vi "Scale Image.vi"(0 "ImageHandler in":refnum<class "ImageHandler.lvclass">, 5 "ImageIn":T1, 7 "Scale?":bool, 11 "error in":errorcluster, 12 "Max":i32, 13 "Min":i32) -> (4 "ImageHandler out":refnum<class "ImageHandler.lvclass">, 6 "ImageOut":T1, 15 "error out":errorcluster)   [LabVIEW 2022 SP3, in "ImageHandler.lvlib" / "ImageHandler.lvclass"]
uses:
  ImageHandler.lvclass
  <vilib>/vision/Image Controls.llb/IMAQ Image.ctl
  ImageHandler.lvclass/ImageHandler.ctl
  <vilib>/vision/NI_Vision_Development_Module.lvlib
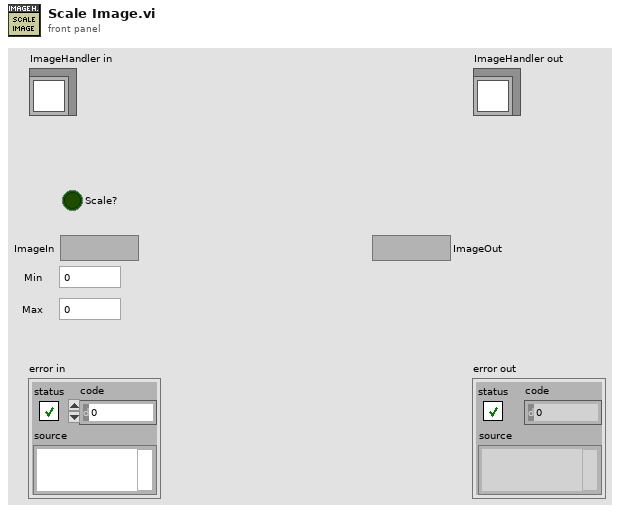
[diagram p1: front panel]
types:
  T1 = typedef "IMAQ Image.ctl" = refnum<image>
  T2 = typedef "Image Type" = u32
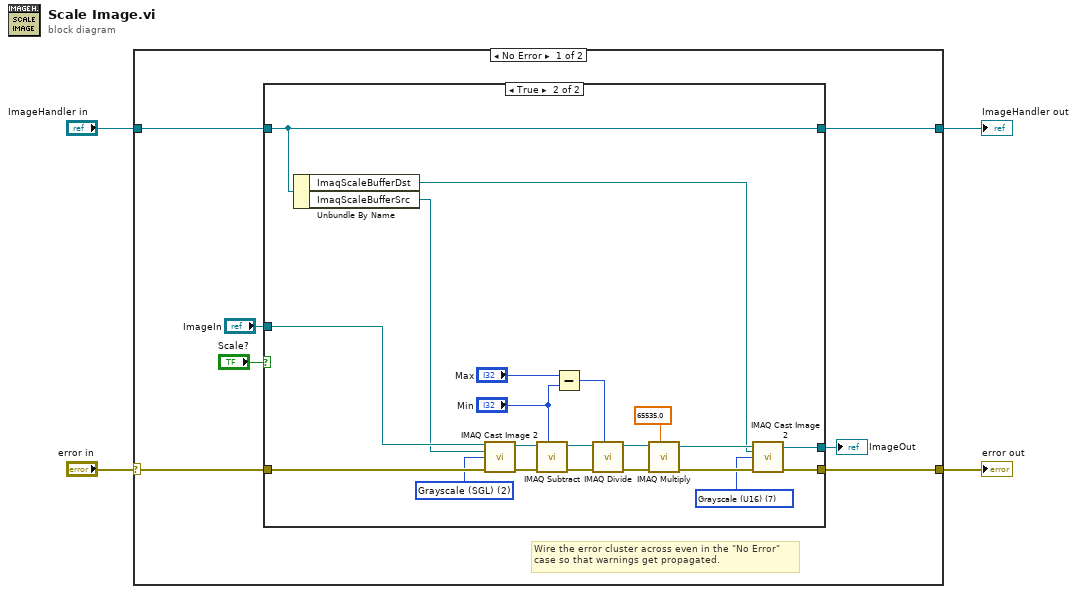
[diagram p0: block diagram]
diagram:
  n1 = case shown="No Error" "error in" {
    selector: "error in" -> [w7 w37]
    tunnel: [w6 w37] -> w3
    tunnel: [w9 w36] -> w1
    tunnel: "ImageHandler in" -> [w10 w36]
    frame No Error {
      # "Wire the error cluster across even in the \"No Error\"\ncase so that warnings get propagated."
      n2 = case shown="True" "Scale?" {
        tunnel: "ImageIn" -> [w13 w33]
        tunnel: w10 -> [w14 w17]
        tunnel: [w14 w17] -> w9
        tunnel: [w13 w18] -> w8
        tunnel: w7 -> [w12 w35]
        tunnel: [w12 w21] -> w6
        frame False {
        }
        frame True {
          w19 = T2 7 items=["Grayscale (U8)", "Grayscale (I16)", "Grayscale (SGL)", "Complex (CSG)", "RGB (U32)", "HSL (U32)", "RGB (U64)", "Grayscale (U16)"] ("Image Type")
          w32 = T2 2 items=["Grayscale (U8)", "Grayscale (I16)", "Grayscale (SGL)", "Complex (CSG)", "RGB (U32)", "HSL (U32)", "RGB (U64)", "Grayscale (U16)"] ("Image Type")
          n3 = Unbundle By Name(w17) -> ("ImaqScaleBufferDst"=w15:T1, "ImaqScaleBufferSrc"=w16:T1)
          n4 = call "IMAQ Cast Image 2"("Image Src"=w33, "Image Dst"=w16, "Image Type"=w32, "error in (no error)"=w35) -> ("Image Dst Out"=w29:T1, "error out"=w34:errorcluster)  [unwired: 10 in]
          n5 = call "IMAQ Subtract"("Image Src A"=w29, "Constant"="Min", "error in (no error)"=w34) -> ("Image Dst Out"=w28:T1, "error out"=w31:errorcluster)  [unwired: 4 in]
          n6 = Subtract(x="Max", y="Min") -> (x-y=w25:i32)
          n7 = call "IMAQ Divide"("Image Src A"=w28, "Constant"=w25, "error in (no error)"=w31) -> ("Image Dst Out"=w22:T1, "error out"=w30:errorcluster)  [unwired: 4 in]
          n8 = call "IMAQ Multiply"("Image Src A"=w22, "Constant"=65535.0, "error in (no error)"=w30) -> ("Image Dst Out"=w20:T1, "error out"=w24:errorcluster)  [unwired: 4 in]
          n9 = call "IMAQ Cast Image 2"("Image Src"=w20, "Image Dst"=w15, "Image Type"=w19, "error in (no error)"=w24) -> ("Image Dst Out"=w18:T1, "error out"=w21:errorcluster)  [unwired: 10 in]
        }
      }
      "ImageOut" <- w8
    }
    frame Error {
    }
  }
  "error out" <- w3
  "ImageHandler out" <- w1
